vi "Read configure scan engine.vi"(8 "error in (no error)":errorcluster, 11 "Scan Engine configuration1 in":refnum<class "Scan Engine configuration.lvclass">) -> (0 "error out":errorcluster, 2 "configure scan engine":bool=TRUE, 3 "Scan Engine configuration1 out":refnum<class "Scan Engine configuration.lvclass">)   [LabVIEW 2015, in "Scan Engine configuration.lvclass"]
uses:
  Scan Engine configuration.lvclass
  Scan Engine configuration.lvclass/Scan Engine configuration.ctl
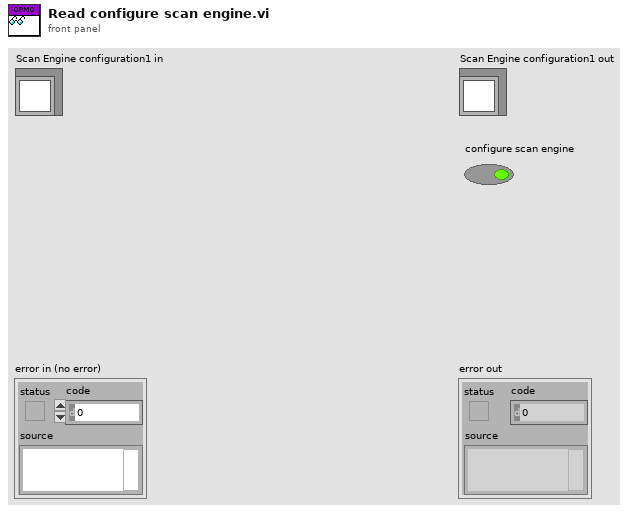
[diagram p1: front panel]
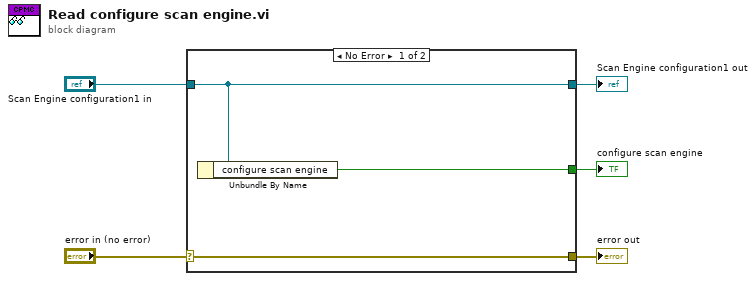
[diagram p0: block diagram]
diagram:
  n1 = case shown="No Error" "error in (no error)" {
    selector: "error in (no error)" -> [w8 w9]
    tunnel: [w8 w9] -> w4
    tunnel: [w7 w10] -> w2
    tunnel: "Scan Engine configuration1 in" -> [w7 w10]
    tunnel: [w6 _] -> w1
    frame No Error {
      n2 = Unbundle By Name(w7) -> ("configure scan engine"=w6:bool)
    }
    frame Error {
    }
  }
  "error out" <- w4
  "Scan Engine configuration1 out" <- w2
  "configure scan engine" <- w1
